vi "PixelReg ProgramFromFile 2nPas.vi"(0 "connection ID":refnum<k5>, 1 "ACQ PxReg folder":path, 2 "EQ folder path":string, 3 "PixelReg (hex)":u32[](array[numeric])=[671965161, 384, 671965161, 384, 671965161, 384, 671965161, 384, 671965161, 384, 671965161, 384, 671965161, 384, 671965161, 384, 671965161, 384, 671965161, 384, 671965161, 384, 671965161, 384, 671965161, 384, 671965161, 384, 671965161, 384, 671965161, 384, 671965161, 384, 671965161, 384, 671965161, 384, 671965161, 384, 671965161, 384, 671965161, 384, 671965161, 384, 671965161, 384, 671965161, 384, 671965161, 384, 671965161, 384, 671965161, 384, 671965161, 384, 671965161, 384, 671965161, 384, 671965161, 384, 671965161, 384, 671965161, 384, 671965161, 384, 671965161, 384, 671965161, 384, 671965161, 384, 671965161, 384, 671965161, 384, 671965161, 384, 671965161, 384, 671965161, 384, 671965161, 384, 671965161, 384, 671965161, 384, 671965161, 384, 671965161, 384, 671965161, 384, 671965161, 384, 671965161, 384, 671965161, 384, 671965161, 384, 671965161, 384, 671965161, 384, 671965161, 384, 671965161, 384, 671965161, 384, 671965161, 384, 671965161, 384, 671965161, 384, 671965161, 384, 671965161, 384, 671965161, 384, 671965161, 384, 671965161, 384, 671965161, 384, 671965161, 384, 671965161, 384, 671965161, 384, 671965161, 384, 671965161, 384, 671965161, 384, 671965161, 384, 671965161, 384, 671965161, 384, 671965161, 384, 671965161, 384, 671965161, 384, 671965161, 384, 671965161, 384, 671965161, 384, 671965161, 384, 671965161, 384, 671965161, 384, 671965161, 384, 671965161, 384, 671965161, 384, 671965161, 384, 671965161, 384, 671965161, 384, 671965161, 384, 671965161, 384, 671965161, 384, 671965161, 384, 671965161, 384, 671965161, 384, 671965161, 384, 671965161, 384, 671965161, 384] format="%x", 5 "All ID list":u32[](array[numeric]) format="%x", 7 "Layer ID list":u32[](array[numeric]) format="%x", 9 "Chip ID list":u32[](array[numeric]) format="%x", 11 "error in (no error)":errorcluster, 12 "PA gain":u8 max=3, 13 "Itest parameter":cluster{"Itest tipus":bool, "I test":u8}={"Itest tipus"=FALSE, "I test"=1} caption="I test parameter" {"I test" max=63 step=1}, 14 "TP EN":bool) -> (4 "connection ID out":refnum<k5>, 6 "done message":string, 8 "quants arxius fets":i32, 10 "All checks OK":bool, 15 "error out (no error)":errorcluster)   [LabVIEW 2015, in "VIPM2.lvlib"]
doc: "Inclou neutralització del ChipID D9EB px14 per ser pixel dolent.\nInclou edició de PA gain i Itest just abans de programar."
uses:
  VIPM2.lvlib
panel:
  out "Progress Bar":sgl(slide) scale=0.0..100.0
  out "iteration":i32
  # "Programming Pixel Registers from files..."
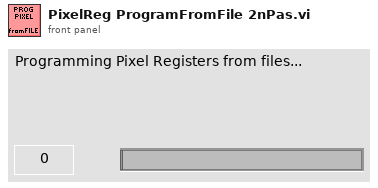
[diagram p1: front panel]
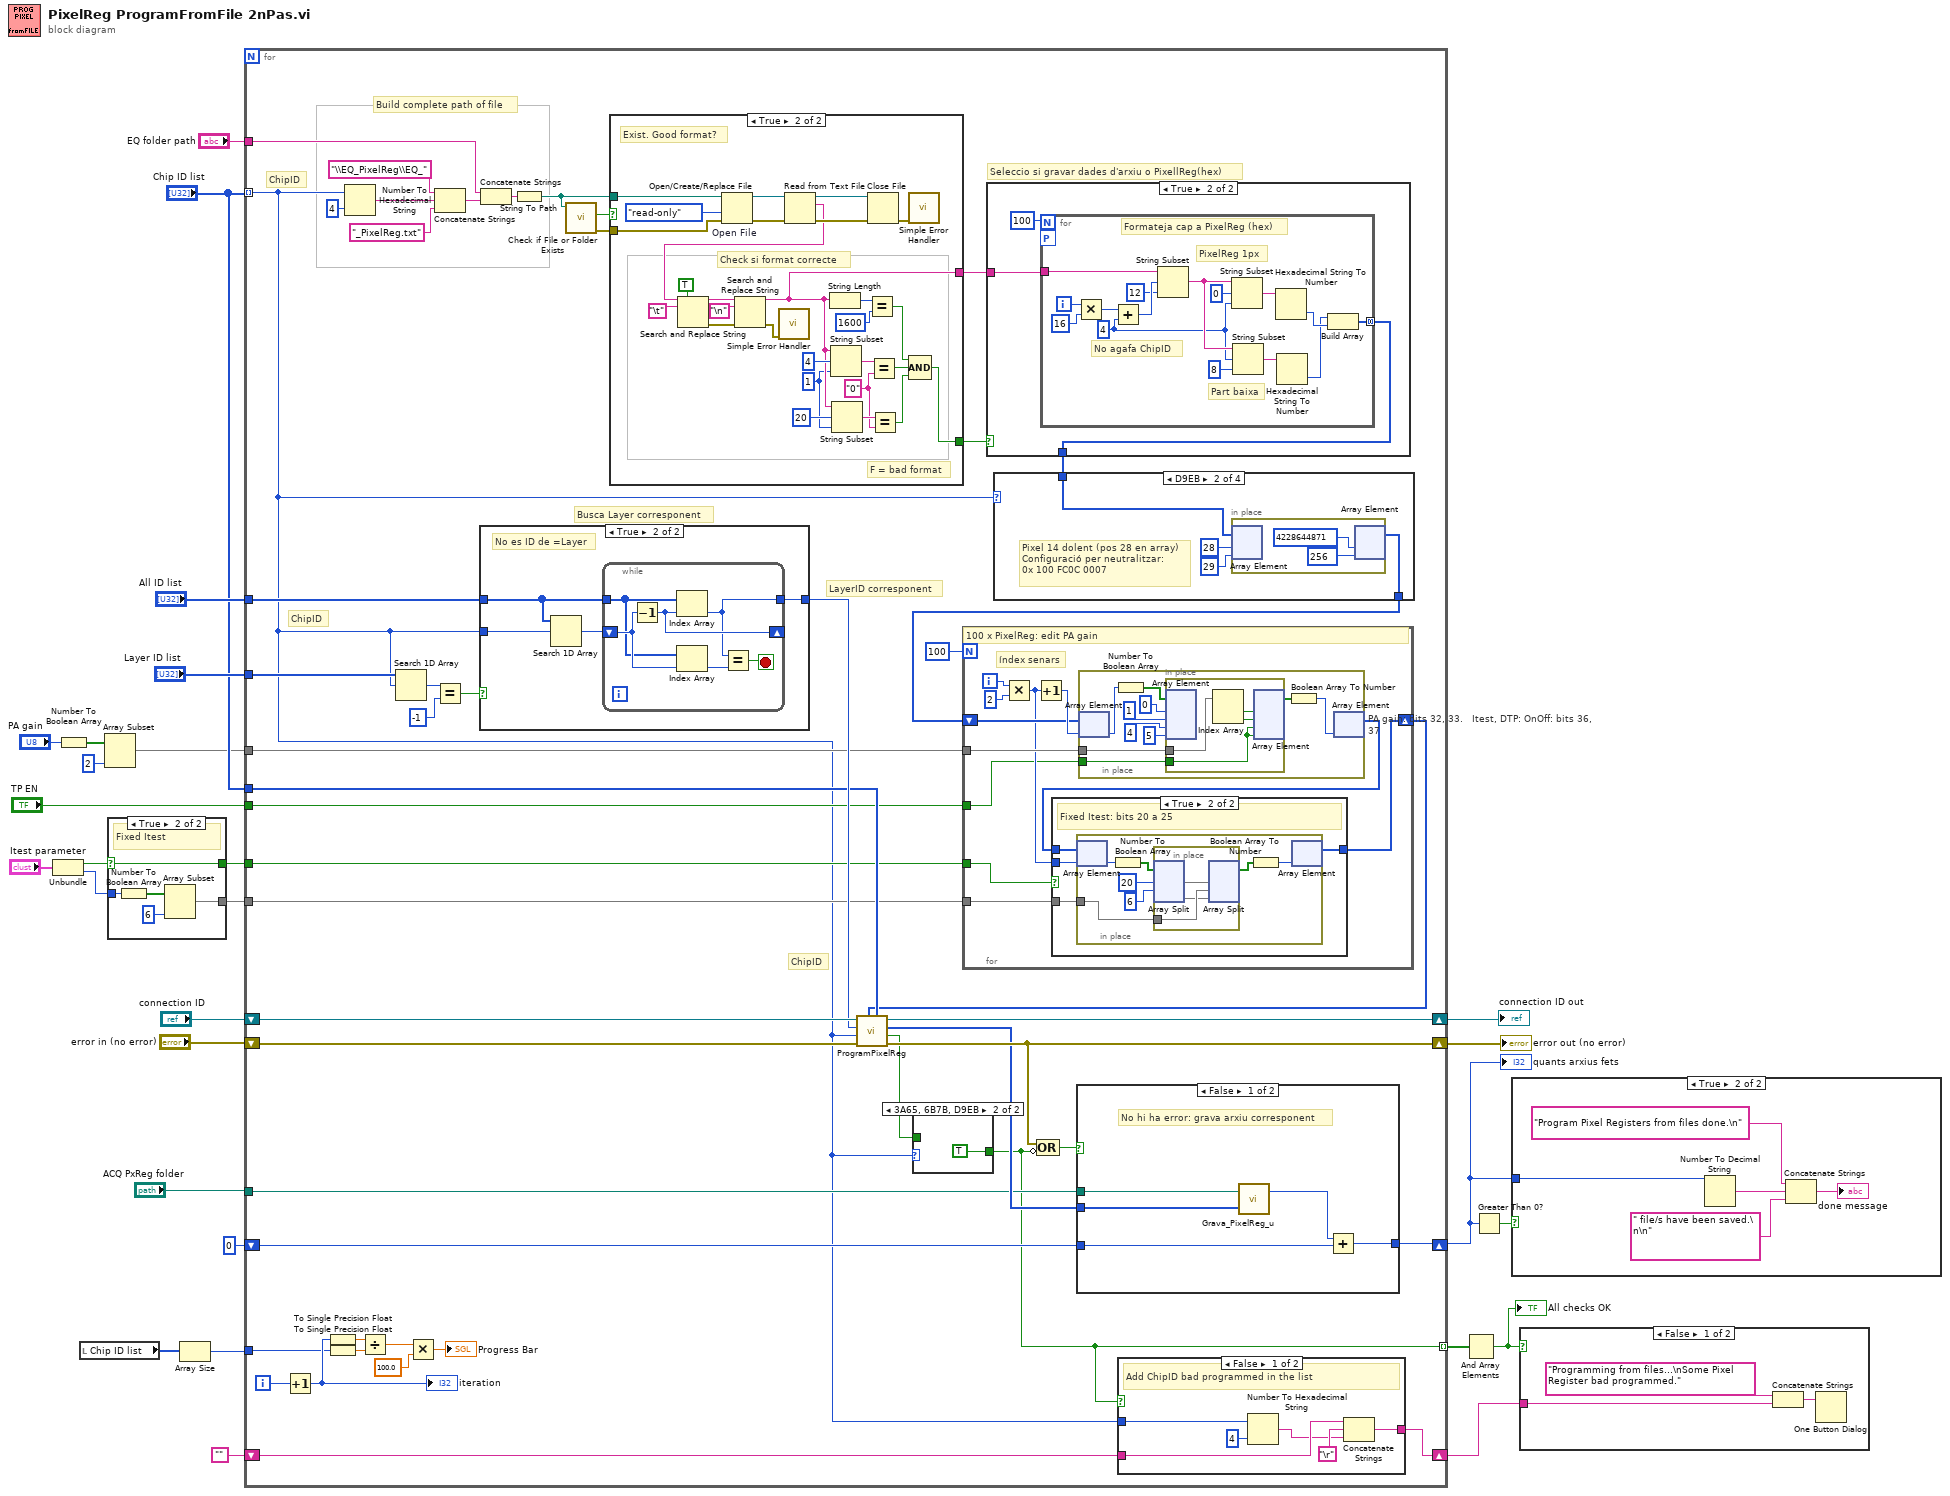
[diagram p0: block diagram]
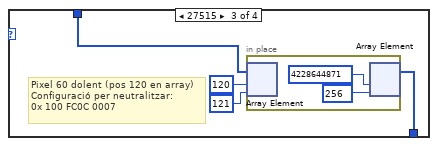
[diagram p9: hidden frame]
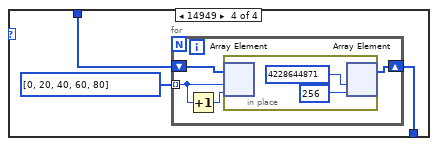
[diagram p10: hidden frame]
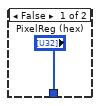
[diagram p13: hidden frame]
diagram:
  n1 = Unbundle("Itest parameter") -> ("Itest tipus"=w5:bool, "I test"=w3:u8)
  n2 = Number To Boolean Array(number="PA gain") -> (Boolean array=w9:bool[])
  n3 = local read "Chip ID list"() -> (w19:u32[])
  n4 = Array Subset "Array Subset"(array=w9, length=2) -> (w7:bool[])  [unwired: 1 in]
  n5 = case shown="True" w5 {
    selector: w5 -> [w29 w32]
    tunnel: [w29 w32] -> w4
    tunnel: w3 -> [_ w31]
    tunnel: [_ w30] -> w2
    frame False {
      # "EQ'd Itest"
    }
    frame True {
      # "Fixed Itest"
      n6 = Number To Boolean Array(number=w31) -> (Boolean array=w33:bool[])
      n7 = Array Subset "Array Subset"(array=w33, length=6) -> (w30:bool[])  [unwired: 1 in]
    }
  }
  n8 = Array Size(array=w19) -> (size(s)=w18:i32)
  n9 = for {
    tunnel: "Chip ID list" -> [w36] mode=indexing
    shift-right: [w64] -> w25
    shift-left: "error in (no error)" -> [w65]
    tunnel: [w35] -> w24 mode=indexing
    shift-right: [w71] -> w20
    shift-left: 0 -> [w70]
    tunnel: w18 -> [w47]
    tunnel: "EQ folder path" -> [w56]
    tunnel: "Layer ID list" -> [w55]
    tunnel: "All ID list" -> [w54]
    tunnel: "ACQ PxReg folder" -> [w53]
    tunnel: "Chip ID list" -> [w51]
    shift-right: [w62] -> w26
    shift-left: "connection ID" -> [w63]
    shift-right: [w46] -> w11
    shift-left: "" -> [w45]
    tunnel: w7 -> [w42]
    tunnel: w4 -> [w41]
    tunnel: w2 -> [w40]
    tunnel: "TP EN" -> [w39]
    i -> [w69]
    # "ChipID"
    # "Busca Layer corresponent"
    # "ChipID"
    # "LayerID corresponent"
    # "ChipID"
    # "Seleccio si gravar dades d'arxiu o PixellReg(hex)"
    # "Build complete path of file"
    n10 = Increment(x=w69) -> (x+1=w49:i32)
    "iteration" <- w49
    n11 = To Single Precision Float(number=w49) -> (single precision float=w50:sgl)
    n12 = To Single Precision Float(number=w47) -> (single precision float=w48:sgl)
    n13 = Number To Hexadecimal String(1:i16 4 ("width (-)"), 2:w36) -> (0:w81:string)
    n14 = Divide(x=w50, y=w48) -> (x/y=w67:sgl)
    n15 = Search 1D Array(1D array=w55, element=w36) -> (index of element=w59:i32)  [unwired: 1 in]
    n16 = Multiply(x=w67, y=sgl 100.0) -> (x*y=→"Progress Bar":sgl)
    n17 = Concatenate Strings("\\EQ_PixelReg\\EQ_" ("string"), w81, "_PixelReg.txt" ("string")) -> (w79:string)
    n18 = Equal?(x=w59, y=-1) -> (x = y?=w57:bool)
    n19 = case shown="True" w57 {
      tunnel: w36 -> [w155 w158]
      tunnel: [w155 w157] -> w61
      tunnel: w54 -> [_ w156]
      frame False {
      }
      frame True {
        # "No es ID de =Layer"
        n20 = Search 1D Array(1D array=w156, element=w158) -> (index of element=w159:i32)  [unwired: 1 in]
        n21 = while {
          tunnel: w156 -> [w164]
          shift-right: [w163] -> _
          shift-left: w159 -> [w165]
          tunnel: [w160] -> w157
          stop <- w161 stop-if-true
          n22 = Decrement(x=w165) -> (x-1=w163:i32)
          n23 = Index Array(array=w164, index=w163) -> (element=w160:u32)
          n24 = Index Array(array=w164, index=w165) -> (element=w162:u32)
          n25 = Equal?(x=w160, y=w162) -> (x = y?=w161:bool)
        }
      }
    }
    n26 = Concatenate Strings(w56, w79) -> (w78:string)
    n27 = String To Path(string=w78) -> (path=w75:path)
    n28 = call <vilib>:"Check if File or Folder Exists.vi"("path"=w75) -> ("error out"=w76:errorcluster, "file or folder exists?"=w77:bool)  [unwired: 8 in, 1 out]
    n29 = case shown="True" w77 {
      selector: w77 -> [w191 _]
      tunnel: w76 -> [_ w197]
      tunnel: [w191 w196] -> w74
      tunnel: w75 -> [_ w198]
      tunnel: [_ w194] -> w73
      frame False {
        # "F = not exist"
        # "File do not exist"
      }
      frame True {
        w193 = "0"
        w192 = 1 ("length (rest)")
        # "F = bad format"
        # "Check si format correcte"
        # "Exist. Good format?"
        n30 = Open/Create/Replace File "Open File"(file path (use dialog)=w198, error in=w197, access (0:read/write)=enum16{"read/write", "read-only", "write-only"}."read-only") -> (refnum out=w200:refnum<file>, error out=w199:errorcluster)  [unwired: 3 in, 1 out]
        n31 = Read from Text File(file (use dialog)=w200, error in=w199) -> (refnum out=w217:refnum<file>, text=w195:string, error out=w218:errorcluster)  [unwired: 2 in, 1 out]
        n32 = Search and Replace String(replace all?=TRUE ("replace all? (F)"), input string=w195, search string="\t") -> (result string=w213:string, error out=w212:errorcluster)  [unwired: 5 in, 2 out]
        n33 = Search and Replace String(input string=w213, search string="\n", error in=w212) -> (result string=w194:string, error out=w210:errorcluster)  [unwired: 5 in, 2 out]
        n34 = call <vilib>:"Simple Error Handler.vi"("error in (no error)"=w210) -> ()  [unwired: 4 in, 5 out]
        n35 = String Length(string=w194) -> (length=w209:i32)
        n36 = String Subset(string=w194, offset (0)=4, length (rest)=w192) -> (substring=w205:string)
        n37 = String Subset(string=w194, offset (0)=20, length (rest)=w192) -> (substring=w201:string)
        n38 = Equal?(x=w209, y=1600) -> (x = y?=w203:bool)
        n39 = Close File(refnum=w217, error in=w218) -> (error out=w214:errorcluster)  [unwired: 1 out]
        n40 = Equal?(x=w205, y=w193) -> (x = y?=w204:bool)
        n41 = Equal?(x=w201, y=w193) -> (x = y?=w202:bool)
        n42 = call <vilib>:"Simple Error Handler.vi"("error in (no error)"=w214) -> ()  [unwired: 4 in, 5 out]
        n43 = Compound Arithmetic op=AND(w203, w204, w202) -> (w196:bool)
      }
    }
    n44 = case shown="True" w74 {
      tunnel: ["PixelReg (hex)" w173] -> w52
      tunnel: w73 -> [_ w174]
      frame False {
      }
      frame True {
        n45 = for {
          N: 100 -> [_]
          tunnel: w174 -> [w189]
          tunnel: [w176] -> w173 mode=concatenating
          workers-P: _ -> [_]
          i -> [w190]
          w182 = 4 ("y")
          # "Formateja cap a PixelReg (hex)"
          # "Part baixa"
          # "PixelReg 1px"
          # "No agafa ChipID"
          n46 = Multiply(x=w190, y=16) -> (x*y=w187:i32)
          n47 = Add(x=w187, y=w182) -> (x+y=w186:i32)
          n48 = String Subset(string=w189, offset (0)=w186, length (rest)=12 ("length (rest)")) -> (substring=w183:string)
          n49 = String Subset(string=w183, offset (0)=0, length (rest)=w182) -> (substring=w180:string)
          n50 = String Subset(string=w183, offset (0)=w182, length (rest)=8 ("length (rest)")) -> (substring=w179:string)
          n51 = Hexadecimal String To Number(string=w180) -> (number=w178:u32)  [unwired: 2 in, 1 out]
          n52 = Hexadecimal String To Number(string=w179) -> (number=w177:u32)  [unwired: 2 in, 1 out]
          n53 = Build Array(w177, w178) -> (w176:u32[])
        }
      }
    }
    n54 = case shown="D9EB" w36 {
      tunnel: w52 -> [w133 w135 w141 w147]
      tunnel: [w133 w134 w140 w146] -> w43
      frame Default {
      }
      frame 55787 {
        # "Pixel 14 dolent (pos 28 en array)\nConfiguració per neutralitzar:\n0x 100 FC0C 0007"
        n55 = in-place {
          n56 = in-place-array #1(w135, 28, 29) -> ()  [unwired: 2 out]
          n57 = in-place-array #1(u32 4228644871 ("Numeric"), u32 256 ("Numeric")) -> (w134:u32[])  [unwired: 2 out]
        }
      }
      frame 27515 {
        # "Pixel 60 dolent (pos 120 en array)\nConfiguració per neutralitzar:\n0x 100 FC0C 0007"
        n58 = in-place {
          n59 = in-place-array #2(w141, 120, 121) -> ()  [unwired: 2 out]
          n60 = in-place-array #2(u32 4228644871 ("Numeric"), u32 256 ("Numeric")) -> (w140:u32[])  [unwired: 2 out]
        }
      }
      frame 14949 {
        n61 = for {
          tunnel: i32[] [0, 20, 40, 60, 80] -> [w149] mode=indexing
          shift-right: [w151] -> w146
          shift-left: w147 -> [w152]
          n62 = Increment(x=w149) -> (x+1=w150:i32)
          n63 = in-place {
            n64 = in-place-array #3(w152, w149, w150) -> ()  [unwired: 2 out]
            n65 = in-place-array #3(u32 4228644871 ("Numeric"), u32 256 ("Numeric")) -> (w151:u32[])  [unwired: 2 out]
          }
        }
      }
    }
    n66 = for {
      N: 100 -> [_]
      tunnel: w42 -> [w92]
      shift-right: [w88] -> w38
      shift-left: w43 -> [w93]
      tunnel: w41 -> [w87]
      tunnel: w40 -> [w91]
      tunnel: w39 -> [w86]
      i -> [w96]
      # "índex senars"
      # "100 x PixelReg: edit PA gain"
      n67 = Multiply(x=w96, y=2) -> (x*y=w89:i32)
      n68 = Increment(x=w89) -> (x+1=w94:i32)
      n69 = in-place "PA gain: bits 32, 33.   Itest, DTP: OnOff: bits 36, 37" {
        in-place-border: w92 -> [w118]
        in-place-border: w86 -> [w112]
        n70 = in-place-array #4(w93, w94) -> (w121:u32)
        n71 = Number To Boolean Array(number=w121) -> (Boolean array=w115:bool[])
        n72 = in-place {
          in-place-border: w118 -> [w125]
          in-place-border: w112 -> [w122]
          n73 = in-place-array #5(w115, 0, 1, 4, 5) -> ()  [unwired: 4 out]
          n74 = Index Array(array=w125) -> (element #1=w124:bool, element #2=w123:bool)  [unwired: 2 in]
          n75 = in-place-array #5(w124, w123, w122, w122) -> (w117:bool[])  [unwired: 4 out]
        }
        n76 = Boolean Array To Number(Boolean array=w117) -> (number=w116:u32)
        n77 = in-place-array #4(w116) -> (w90:u32[])  [unwired: 1 out]
      }
      n78 = case shown="True" w87 {
        tunnel: w91 -> [_ w99]
        tunnel: w90 -> [w97 w101]
        tunnel: w89 -> [_ w100]
        tunnel: [w97 w98] -> w88
        frame False {
          # "EQ'd Itest"
        }
        frame True {
          # "Fixed Itest: bits 20 a 25"
          n79 = in-place {
            in-place-border: w99 -> [w104]
            n80 = in-place-array #6(w101, w100) -> (w108:u32)
            n81 = Number To Boolean Array(number=w108) -> (Boolean array=w107:bool[])
            n82 = in-place {
              in-place-border: w104 -> [w110]
              n83 = in-place-split #7(w107, 20, 6) -> (w111:bool[], w109:bool[])  [unwired: 1 out]
              n84 = in-place-split #7(w111, w110, w109) -> (w103:bool[])  [unwired: 2 out]
            }
            n85 = Boolean Array To Number(Boolean array=w103) -> (number=w102:u32)
            n86 = in-place-array #6(w102) -> (w98:u32[])  [unwired: 1 out]
          }
        }
      }
    }
    n87 = call "ProgramPixelReg.vi"("Chip ID list"=w51, "Pixel Register"=w38, "error in (no error)"=w65, "ChipID"=w36, "LayerID"=w61, "connection ID"=w63) -> ("error out"=w64:errorcluster, "OK?"=w37:bool, "PixelReg programmed"=w60:u32[], "connection ID out"=w62:refnum<k5>)  [unwired: 1 in, 1 out]
    n88 = case shown="3A65, 6B7B, D9EB" w36 {
      tunnel: w37 -> [w84 _]
      tunnel: [w84 TRUE] -> w35
      frame Default {
      }
      frame 14949, 27515, 55787 {
      }
    }
    n89 = Compound Arithmetic op=OR(w64, invert w35) -> (w72:bool)
    n90 = case shown="False" w72 {
      tunnel: w60 -> [w168 _]
      tunnel: [w170 w171] -> w71
      tunnel: w70 -> [w169 w171]
      tunnel: w53 -> [w166 _]
      frame False {
        # "No hi ha error: grava arxiu corresponent"
        n91 = call "Grava_PixelReg_u.vi"("Pixel Register programmed"=w168, "Folder path"=w166) -> ("quants arxius fets"=w167:i32)  [unwired: 1 in]
        n92 = Add(x=w167, y=w169) -> (x+y=w170:i32)
      }
      frame True {
        # "Hi ha algun error"
      }
    }
    n93 = case shown="False" w35 {
      tunnel: w36 -> [w131 _]
      tunnel: [w129 w132] -> w46
      tunnel: w45 -> [w128 w132]
      frame False {
        # "Add ChipID bad programmed in the list"
        n94 = Number To Hexadecimal String(1:i16 4 ("width (-)"), 2:w131) -> (0:w126:string)
        n95 = Concatenate Strings(w128, "\r", w126) -> (w129:string)
      }
      frame True {
      }
    }
  }
  "connection ID out" <- w26
  "error out (no error)" <- w25
  "quants arxius fets" <- w20
  n96 = And Array Elements(Boolean array=w24) -> (logical AND=w23:bool)
  "All checks OK" <- w23
  n97 = Greater Than 0?(x=w20) -> (x > 0?=w21:bool)
  n98 = case shown="True" w21 {
    tunnel: w20 -> [_ w222]
    frame False {
    }
    frame True {
      n99 = Number To Decimal String(number=w222) -> (decimal integer string=w224:string)  [unwired: 1 in]
      n100 = Concatenate Strings("Program Pixel Registers from files done.\n" ("string"), w224, " file/s have been saved.\n\n") -> (→"done message":string)
    }
  }
  n101 = case shown="False" w23 {
    tunnel: w11 -> [w225 _]
    frame False {
      n102 = Concatenate Strings("Programming from files...\nSome Pixel Register bad programmed." ("message"), w225) -> (w227:string)
      n103 = One Button Dialog(message=w227) -> ()  [unwired: 1 in, 1 out]
    }
    frame True {
      # "All checks OK"
    }
  }
